vi "LogSave.vi"(0 "GenericCanAdapterClass in":refnum<class "GenericCanAdapterClass.lvclass">, 11 "error in":errorcluster) -> (4 "GenericCanAdapterClass out":refnum<class "GenericCanAdapterClass.lvclass">, 15 "error out":errorcluster)   [LabVIEW 2011, in "GenericCanAdapterClass.lvclass"]
uses:
  GenericCanAdapterClass.lvclass
  GenericCanAdapterClass.lvclass/GenericCanAdapterClass.ctl
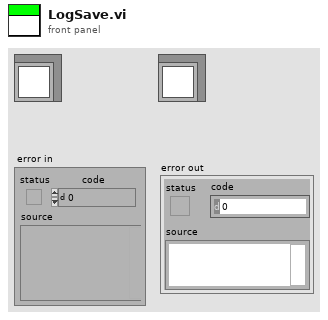
[diagram p1: front panel]
types:
  T1 = enum16{"open", "replace", "create", "open or create", "replace or create", "replace or create with confirmation"}
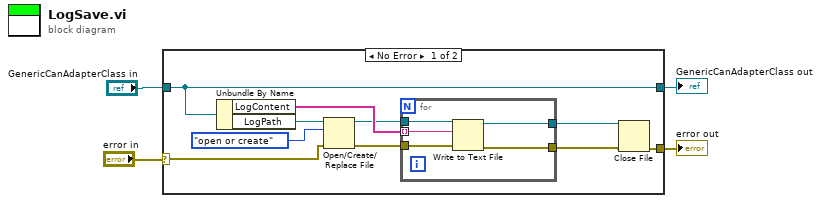
[diagram p0: block diagram]
diagram:
  n1 = case shown="No Error" "error in" {
    selector: "error in" -> [w6 w21]
    tunnel: "GenericCanAdapterClass in" -> [w5 w20]
    tunnel: [w7 w21] -> w3
    tunnel: [w5 w20] -> w1
    frame No Error {
      n2 = Unbundle By Name(w5) -> ("LogContent"=w12:string[], "LogPath"=w14:path)
      n3 = Open/Create/Replace File(file path (use dialog)=w14, error in=w6, operation (0:open)=T1."open or create") -> (refnum out=w8:refnum<file>, error out=w11:errorcluster)  [unwired: 3 in, 1 out]
      n4 = for {
        tunnel: w12 -> [w19] mode=indexing
        tunnel: w11 -> [w18]
        tunnel: [w17] -> w10
        tunnel: [w16] -> w9
        tunnel: w8 -> [w15]
        n5 = Write to Text File(file (use dialog)=w15, text=w19, error in=w18) -> (refnum out=w16:refnum<file>, error out=w17:errorcluster)  [unwired: 1 in, 1 out]
      }
      n6 = Close File(refnum=w9, error in=w10) -> (error out=w7:errorcluster)  [unwired: 1 out]
    }
    frame Error {
    }
  }
  "error out" <- w3
  "GenericCanAdapterClass out" <- w1
